vi "Teleop.vi"(10 "Match Info":T1={"Autonomous Elapsed Seconds"=0.0, "TeleOp Elapsed Seconds"=0.0, "Disabled Elapsed Seconds"=0.0, "Visited Autonomous"=FALSE, "Visited TeleOp"=FALSE, "Visited Disabled"=FALSE, "Autonomous Settings"={"Autonomous Style"=enum."Independent", "VI Refnum"=refnum}}, 11 "Call Context":T2) -> ()   [LabVIEW 2015]
doc: "This VI is called for each TeleOp packet received from the DS where the robot is not disabled. It is often used to read from the joysticks and update I/O or to update setpoints for timed control loops. It should complete and return within 20 milliseconds or it may miss DS packets."
uses:
  <vilib>/Rock Robotics/WPI/DriverStation/WPI_DriverStationDerivedRobotMode.ctl
  <vilib>/Rock Robotics/WPI/DriverStation/WPI_DriverStationMatch Info.ctl
  <vilib>/Rock Robotics/WPI/Solenoid/WPI_SolenoidValue.ctl
  <vilib>/Rock Robotics/WPI/Utilities/WPI_GetSetVariantRefNum.vi
  Robot Global Data.vi
  <vilib>/Rock Robotics/Network Tables/NT Write Boolean.vi
  <vilib>/Rock Robotics/Network Tables/NT Write Numeric Array.vi
  <vilib>/Rock Robotics/Network Tables/NT Read Boolean.vi
  <vilib>/Rock Robotics/Network Tables/NT Read Number.vi
  <vilib>/Rock Robotics/WPI/Solenoid/WPI_SolenoidSetEnum.vi
panel:
  out "Sample Slider 0":dbl(slide) scale=0.0..5.0
  out "Sample Boolean 1":bool
  out "Sample Boolean 0":bool
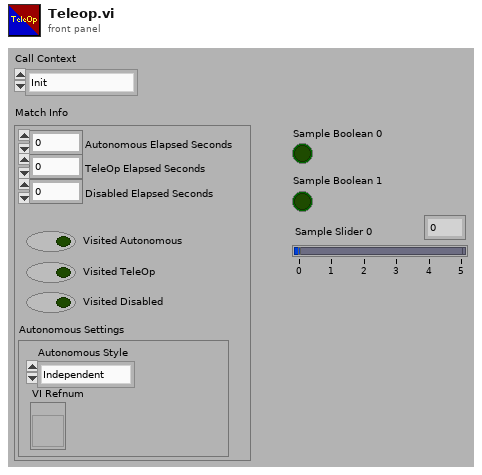
[diagram p1: front panel]
types:
  T1 = typedef "WPI_DriverStationMatch Info.ctl" = cluster{"Autonomous Elapsed Seconds":dbl, "TeleOp Elapsed Seconds":dbl, "Disabled Elapsed Seconds":dbl, "Visited Autonomous":bool, "Visited TeleOp":bool, "Visited Disabled":bool, "Autonomous Settings":cluster{"Autonomous Style":enum16{"Iterative", "Independent"}, "VI Refnum":refnum<vi>}}
  T2 = typedef "WPI_DriverStationDerivedRobotMode.ctl" = enum16{"Init", "Execute", "Stop"}
  T3 = typedef "WPI_SolenoidValue.ctl" = enum16{"Off", "On", "Forward", "Reverse"}
  T4 = typedef "WPI_JoystickDevRef.ctl" = cluster{"Device":T5}
  T5 = typedef "WPI_JoystickDeviceEnum.ctl" = enum16{"USB 0", "USB 1", "USB 2", "USB 3", "USB 4", "USB 5"}
  T6 = cluster{"Buttons[0]":bool, "Buttons[1]":bool, "Buttons[2]":bool, "Buttons[3]":bool, "Buttons[4]":bool, "Buttons[5]":bool, "Buttons[6]":bool, "Buttons[7]":bool, "Buttons[8]":bool}
  T7 = typedef "WPI_DigitalInputDevRef.ctl" = cluster{"DevStatus":errorcluster, "DIO Channel":T8}
  T8 = typedef "FPGA_DIOChannel.ctl" = enum8{"DIO 0", "DIO 1", "DIO 2", "DIO 3", "DIO 4", "DIO 5", "DIO 6", "DIO 7", "DIO 8", "DIO 9", "DIO MXP 0", "DIO MXP 1", "DIO MXP 2", "DIO MXP 3", "DIO MXP 4", "DIO MXP 5", "DIO MXP 6", "DIO MXP 7", "DIO MXP 8", "DIO MXP 9", "DIO MXP 10", "DIO MXP 11", "DIO MXP 12", "DIO MXP 13", "DIO MXP 14", "DIO MXP 15", "Invalid"}
  T9 = typedef "WPI_RobotDriveDevRef.ctl" = cluster{"DevStatus":errorcluster, "Motors[]":T10[], "Square Inputs":bool, "Max Output":dbl}
  T10 = typedef "WPI_MotorControlDeviceRef.ctl" = cluster{"DeviceStatus":errorcluster, "Type":T11, "PWM":cluster{"PWM Channel":T12, "DeadBand":T13}, "CAN":cluster{"Device Number":u8, "Control Mode":T14, "Semaphore":T15, "Max Vout":dbl, "TalonSRX Control Mode":T16}, "Invert":bool}
  T11 = typedef "WPI_MotorControlType.ctl" = enum16{"PWM", "CAN", "CANTalonSRX"}
  T12 = typedef "FPGA_DIOPWMChannel.ctl" = enum8{"PWM 0", "PWM 1", "PWM 2", "PWM 3", "PWM 4", "PWM 5", "PWM 6", "PWM 7", "PWM 8", "PWM 9", "PWM MXP 0", "PWM MXP 1", "PWM MXP 2", "PWM MXP 3", "PWM MXP 4", "PWM MXP 5", "PWM MXP 6", "PWM MXP 7", "PWM MXP 8", "PWM MXP 9", "Invalid"}
  T13 = typedef "WPI_PWMDeadband.ctl" = cluster{"Name":string, "maxPositivePwm":i32, "minPositivePwm":i32, "centerPwm":i32, "maxNegativePwm":i32, "minNegativePwm":i32, "angularRange":u16}
  T14 = typedef "WPI_CANJaguar_ControlMode.ctl" = enum8{"Percent VBus", "Current", "Speed", "Position", "Voltage"}
  T15 = typedef "Semaphore RefNum" = refnum<k1>
  T16 = typedef "WPI_CANTalonSRX_APIControlMode.ctl" = enum8{"Percent VBus", "Speed", "Position", "Slave", "Unchanged / Invalid", "Voltage Compensation", "Current", "Motion Profile"}
  T17 = typedef "WPI_SolenoidDevRef.ctl" = cluster{"DevStatus":errorcluster, "Pneumatics Control Module":u8, "Forward Solenoid Channel":T18, "Reverse Solenoid Channel":T18}
  T18 = typedef "WPI_SolenoidChannel.ctl" = enum8{"Solenoid 0", "Solenoid 1", "Solenoid 2", "Solenoid 3", "Solenoid 4", "Solenoid 5", "Solenoid 6", "Solenoid 7", "Invalid"}
  T19 = typedef "WPI_ServoDeviceRef.ctl" = cluster{"DeviceStatus":errorcluster, "PWM Channel":T12, "DeadBand":T13}
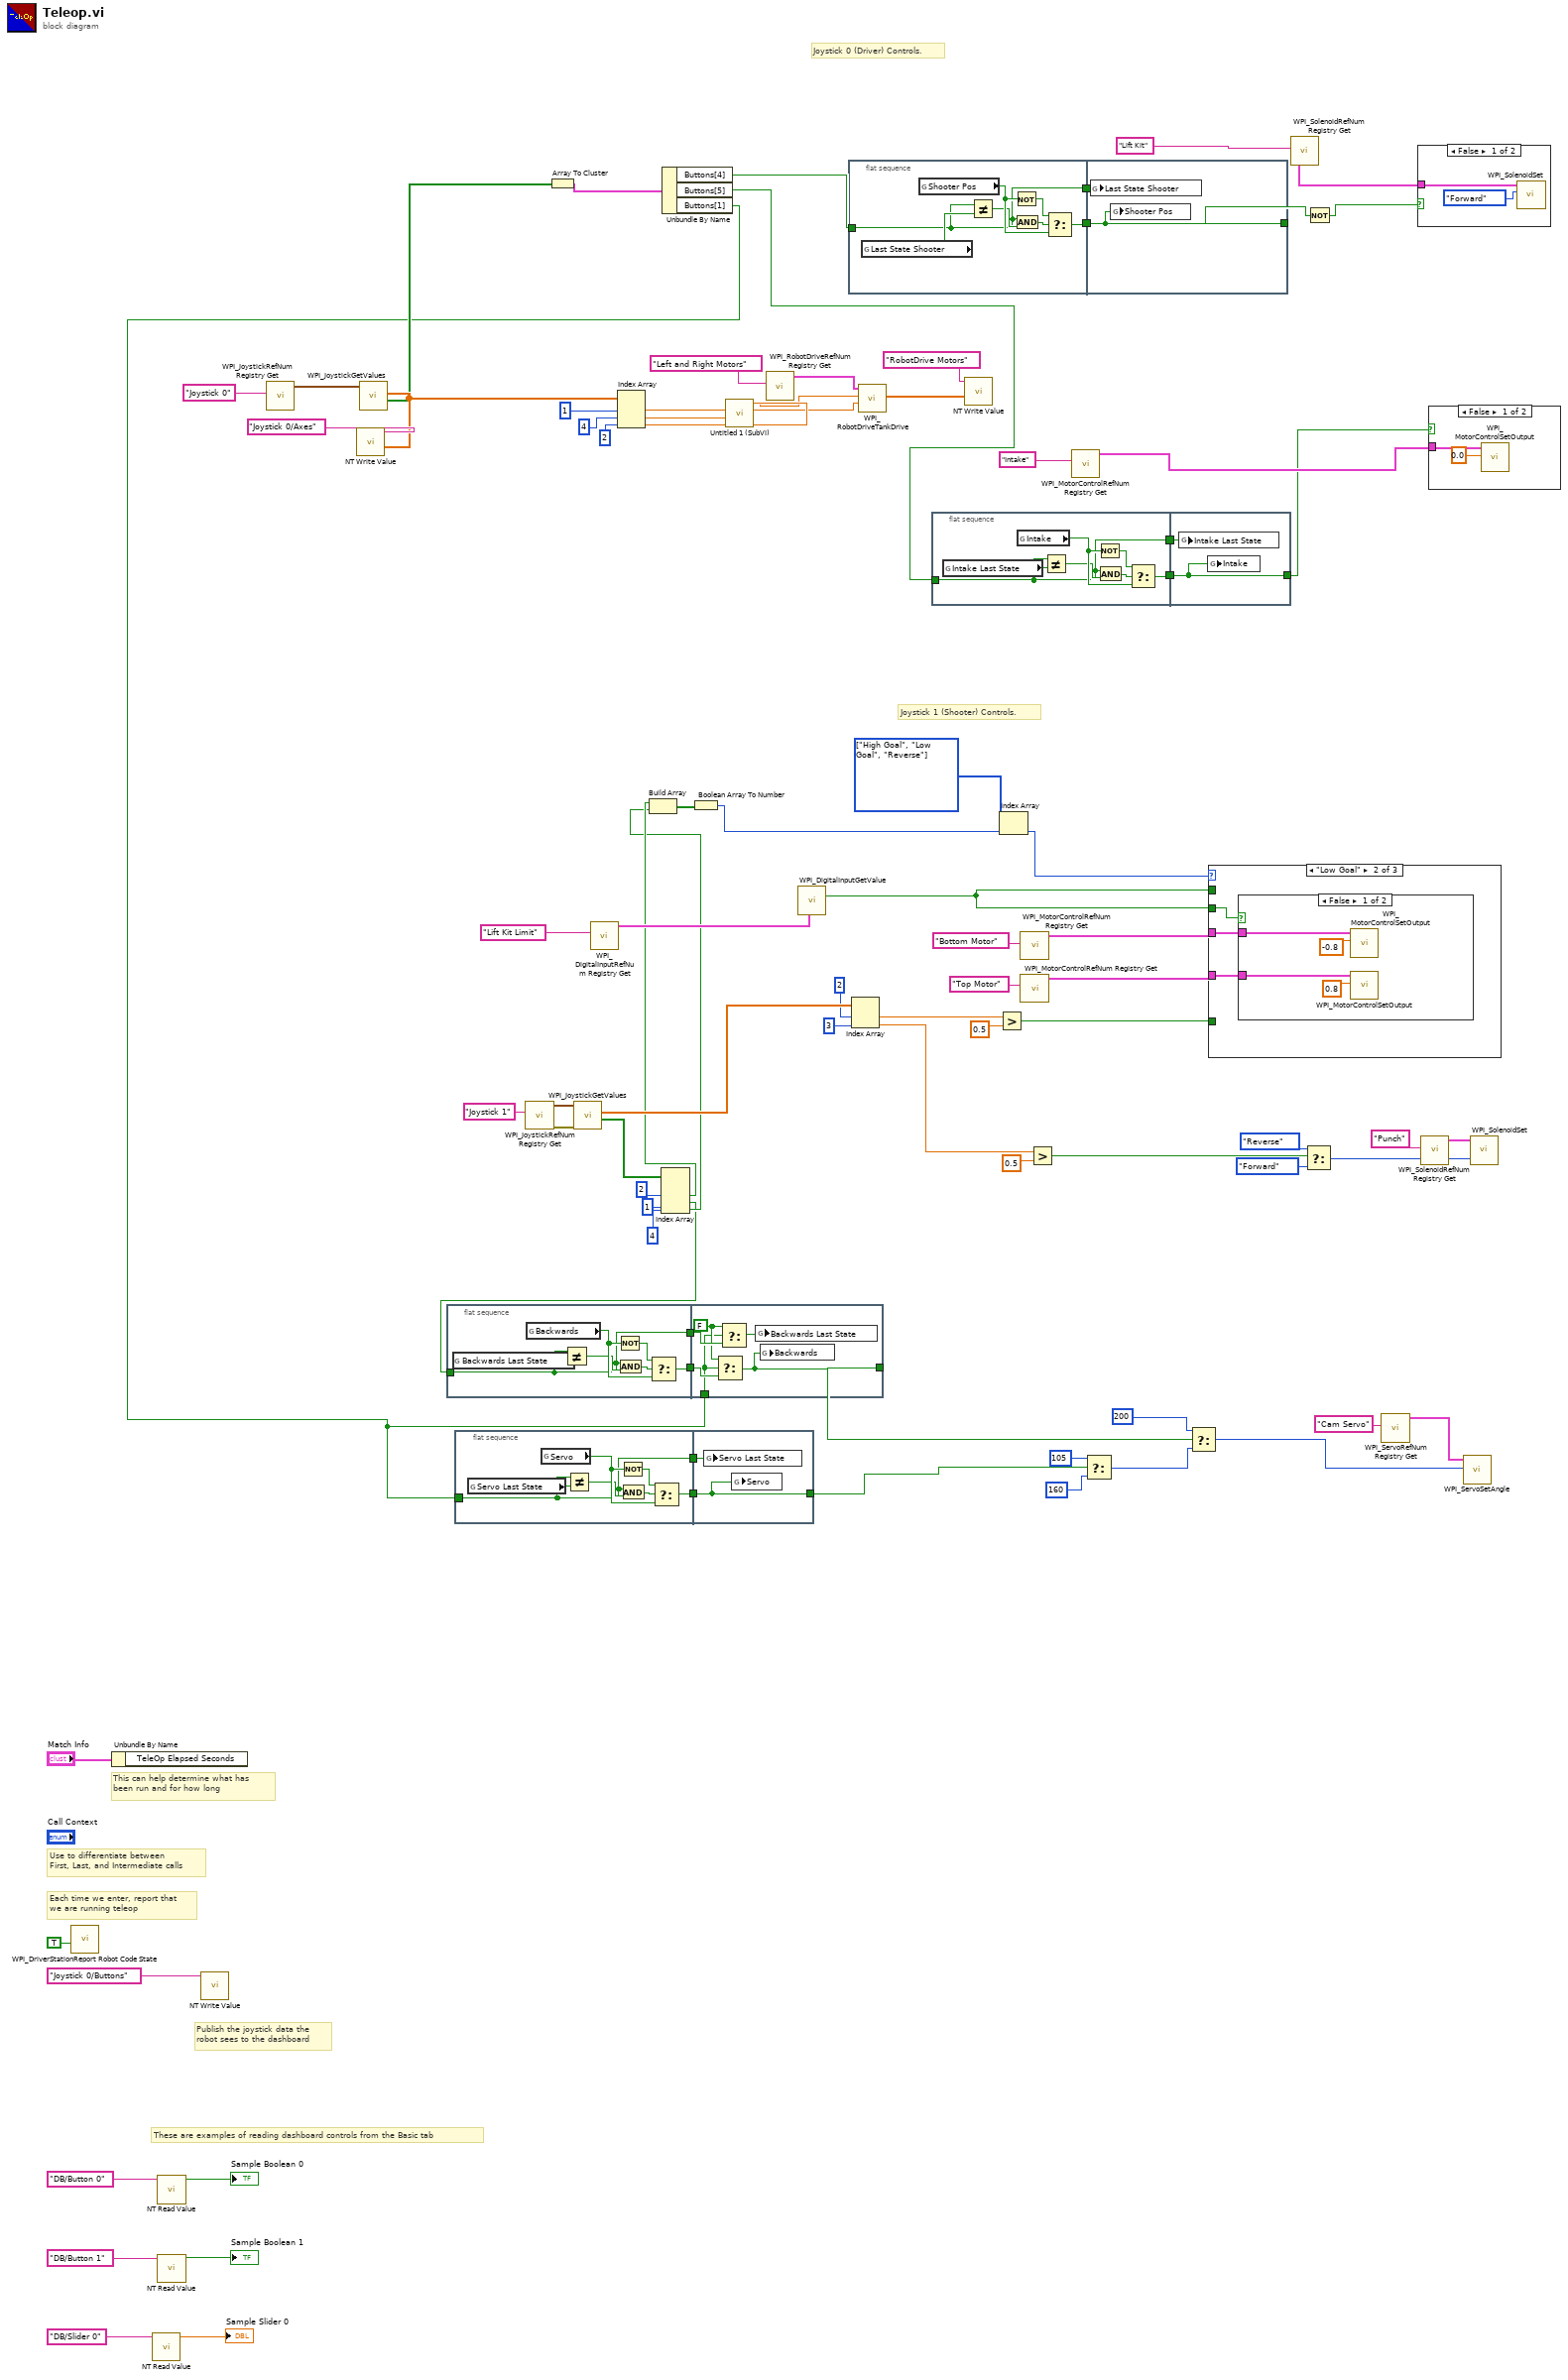
[diagram p0: block diagram]
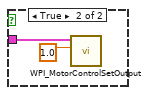
[diagram p2: hidden frame]
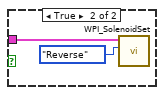
[diagram p3: hidden frame]
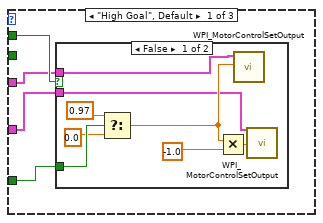
[diagram p4: hidden frame]
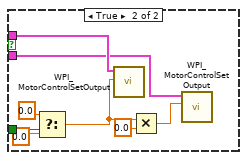
[diagram p5: hidden frame]
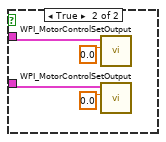
[diagram p6: hidden frame]
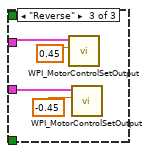
[diagram p7: hidden frame]
diagram:
  w29 = enum16{"High Goal", "Low Goal", "Reverse", ""}[] [enum."High Goal", enum."Low Goal", enum."Reverse"] items=["High Goal", "Low Goal", "Reverse", ""] ("array")
  # "Joystick 1 (Shooter) Controls."
  # "Joystick 0 (Driver) Controls."
  # "These are examples of reading dashboard controls from the Basic tab"
  # "Publish the joystick data the\nrobot sees to the dashboard"
  # "Each time we enter, report that\nwe are running teleop"
  # "Use to differentiate between\nFirst, Last, and Intermediate calls"
  # "This can help determine what has\nbeen run and for how long"
  n1 = call <vilib>:"WPI_DriverStationReport Robot Code State.vi"("TeleOp"=TRUE ("Autonomous")) -> ()  [unwired: 10 in, 1 out]
  n2 = Unbundle By Name("Match Info") -> ()  [unwired: 1 out]
  n3 = call-poly <vilib>:"NT Read Value.vi"("Name"="DB/Slider 0" ("refnum name")) -> ("Numeric"=→"Sample Slider 0":dbl)  [unwired: 9 in, 1 out]
  n4 = call-poly <vilib>:"NT Read Value.vi"("Name"="DB/Button 0" ("refnum name")) -> ("Boolean"=→"Sample Boolean 0":bool)  [unwired: 9 in, 1 out]
  n5 = call-poly <vilib>:"NT Read Value.vi"("Name"="DB/Button 1" ("refnum name")) -> ("Boolean"=→"Sample Boolean 1":bool)  [unwired: 9 in, 1 out]
  n6 = call-poly <vilib>:"NT Write Value.vi"("Name"="Joystick 0/Buttons") -> ()  [unwired: 10 in, 1 out]
  n7 = call <vilib>:"WPI_JoystickRefNum Registry Get.vi"("refnum name"="Joystick 0") -> ("JoystickDevRef"=w87:T4)  [unwired: 1 in, 9 out]
  n8 = call <vilib>:"WPI_JoystickGetValues.vi"("JoystickDevRef"=w87) -> ("Buttons"=w74:bool[], "Axes"=w83:dbl[])  [unwired: 6 in, 3 out]
  n9 = call-poly <vilib>:"NT Write Value.vi"("Numeric Array"=w83, "Name"="Joystick 0/Axes") -> ()  [unwired: 9 in, 1 out]
  n10 = flat-sequence {
    tunnel: w9 -> [w90]
    tunnel: [w94] -> w11
    tunnel: [w90] -> w10
    tunnel: w11 -> [w99]
    tunnel: [w100] -> w8
    tunnel: w10 -> [w101]
    tunnel: w1 -> [w97]
    frame #0 {
      n11 = global read "Robot Global Data.vi" "Backwards Last State"() -> (w93:bool)
      n12 = global read "Robot Global Data.vi" "Backwards"() -> (w95:bool)
      n13 = Not Equal?(x=w90, y=w93) -> (x != y?=w91:bool)
      n14 = Not(x=w95) -> (.not. x?=w96:bool)
      n15 = And(x=w90, y=w91) -> (x .and. y?=w92:bool)
      n16 = Select(t=w96, s=w92, f=w95) -> (s? t:f=w94:bool)
    }
    frame #1 {
      w98 = FALSE ("t")
      n17 = Select(t=w98, s=w97, f=w99) -> (s? t:f=w100:bool)
      n18 = Select(t=w98, s=w97, f=w101) -> (s? t:f=w102:bool)
      n19 = global write "Robot Global Data.vi" "Backwards Last State"(w102) -> ()
      n20 = global write "Robot Global Data.vi" "Backwards"(w100) -> ()
    }
  }
  n21 = flat-sequence {
    tunnel: w1 -> [w103]
    tunnel: [w107] -> w18
    tunnel: [w103] -> w17
    tunnel: w18 -> [w111]
    tunnel: [w111] -> w7
    tunnel: w17 -> [w110]
    frame #0 {
      n22 = global read "Robot Global Data.vi" "Servo Last State"() -> (w106:bool)
      n23 = global read "Robot Global Data.vi" "Servo"() -> (w108:bool)
      n24 = Not Equal?(x=w103, y=w106) -> (x != y?=w104:bool)
      n25 = Not(x=w108) -> (.not. x?=w109:bool)
      n26 = And(x=w103, y=w104) -> (x .and. y?=w105:bool)
      n27 = Select(t=w109, s=w105, f=w108) -> (s? t:f=w107:bool)
    }
    frame #1 {
      n28 = global write "Robot Global Data.vi" "Servo Last State"(w110) -> ()
      n29 = global write "Robot Global Data.vi" "Servo"(w111) -> ()
    }
  }
  n30 = call <vilib>:"WPI_JoystickRefNum Registry Get.vi"("refnum name"="Joystick 1") -> ("error out"=w69:errorcluster, "JoystickDevRef"=w68:T4)  [unwired: 1 in, 8 out]
  n31 = Array To Cluster(array=w74) -> (cluster=w76:T6)
  n32 = call <vilib>:"WPI_JoystickGetValues.vi"("error in (no error)"=w69, "JoystickDevRef"=w68) -> ("Buttons"=w54:bool[], "Axes"=w67:dbl[])  [unwired: 5 in, 3 out]
  n33 = call <vilib>:"WPI_DigitalInputRefNum Registry Get.vi"("refnum name"="Lift Kit Limit") -> ("DigitalInputDevRef"=w57:T7)  [unwired: 9 in, 1 out]
  n34 = Index Array(array=w83, index #1=1 ("index"), index #2=4 ("index"), index #3=2 ("index")) -> (element #1=w61:dbl, element #2=w62:dbl, element #3=w60:dbl)
  n35 = Index Array(array=w54, index #2=2 ("index"), index #3=1 ("index"), index #4=4 ("index")) -> (element #2=w36:bool, element #3=w9:bool, element #4=w35:bool)  [unwired: 1 in, 1 out]
  n36 = Build Array(w36, w35) -> (w27:bool[])
  n37 = Unbundle By Name(w76) -> ("Buttons[4]"=w25:bool, "Buttons[5]"=w19:bool, "Buttons[1]"=w1:bool)
  n38 = Boolean Array To Number(Boolean array=w27) -> (number=w26:u32)
  n39 = call "Untitled 1 (SubVI).vi"("upper limit 2"=w62, "upper limit"=w61, "Throttle"=w60) -> ("Numeric 2"=w47:dbl, "Numeric"=w48:dbl)  [unwired: 7 in]
  n40 = call <vilib>:"WPI_RobotDriveRefNum Registry Get.vi"("refnum name"="Left and Right Motors") -> ("RobotDriveDevRef"=w46:T9)  [unwired: 1 in, 9 out]
  n41 = call <vilib>:"WPI_DigitalInputGetValue.vi"("DigitalInputDevRef"=w57) -> ("Value"=w55:bool)  [unwired: 8 in, 2 out]
  n42 = flat-sequence {
    tunnel: w25 -> [w112]
    tunnel: [w116] -> w24
    tunnel: [w112] -> w23
    tunnel: w24 -> [w120]
    tunnel: [w120] -> w16
    tunnel: w23 -> [w119]
    frame #0 {
      n43 = global read "Robot Global Data.vi" "Last State Shooter"() -> (w115:bool)
      n44 = global read "Robot Global Data.vi" "Shooter Pos"() -> (w117:bool)
      n45 = Not Equal?(x=w112, y=w115) -> (x != y?=w113:bool)
      n46 = Not(x=w117) -> (.not. x?=w118:bool)
      n47 = And(x=w112, y=w113) -> (x .and. y?=w114:bool)
      n48 = Select(t=w118, s=w114, f=w117) -> (s? t:f=w116:bool)
    }
    frame #1 {
      n49 = global write "Robot Global Data.vi" "Last State Shooter"(w119) -> ()
      n50 = global write "Robot Global Data.vi" "Shooter Pos"(w120) -> ()
    }
  }
  n51 = Index Array(array=w67, index #1=2 ("index"), index #2=3 ("index")) -> (element #1=w66:dbl, element #2=w32:dbl)
  n52 = call <vilib>:"WPI_RobotDriveTankDrive.vi"("Right axis value"=w47, "Left axis value"=w48, "RobotDriveDevRef"=w46) -> ("Motor Values"=w71:dbl[])  [unwired: 6 in, 2 out]
  n53 = flat-sequence {
    tunnel: w19 -> [w121]
    tunnel: [w125] -> w22
    tunnel: [w121] -> w21
    tunnel: w22 -> [w129]
    tunnel: [w129] -> w20
    tunnel: w21 -> [w128]
    frame #0 {
      n54 = global read "Robot Global Data.vi" "Intake Last State"() -> (w124:bool)
      n55 = global read "Robot Global Data.vi" "Intake"() -> (w126:bool)
      n56 = Not Equal?(x=w121, y=w124) -> (x != y?=w122:bool)
      n57 = Not(x=w126) -> (.not. x?=w127:bool)
      n58 = And(x=w121, y=w122) -> (x .and. y?=w123:bool)
      n59 = Select(t=w127, s=w123, f=w126) -> (s? t:f=w125:bool)
    }
    frame #1 {
      n60 = global write "Robot Global Data.vi" "Intake Last State"(w128) -> ()
      n61 = global write "Robot Global Data.vi" "Intake"(w129) -> ()
    }
  }
  n62 = call-poly <vilib>:"NT Write Value.vi"("Numeric Array"=w71, "Name"="RobotDrive Motors") -> ()  [unwired: 9 in, 1 out]
  n63 = Greater?(x=w66, y=0.5) -> (0:w65:bool)
  n64 = Index Array(array=w29, index=w26) -> (element=w28:enum16{"High Goal", "Low Goal", "Reverse", ""})
  n65 = call <vilib>:"WPI_MotorControlRefNum Registry Get.vi"("refnum name"="Bottom Motor") -> ("MotorControlDevRef"=w39:T10)  [unwired: 9 in, 1 out]
  n66 = call <vilib>:"WPI_MotorControlRefNum Registry Get.vi"("refnum name"="Top Motor") -> ("MotorControlDevRef"=w38:T10)  [unwired: 9 in, 1 out]
  n67 = Greater?(x=w32, y=0.5) -> (0:w30:bool)
  n68 = call <vilib>:"WPI_MotorControlRefNum Registry Get.vi"("refnum name"="Intake") -> ("MotorControlDevRef"=w50:T10)  [unwired: 9 in, 1 out]
  n69 = Select(t=105, s=w7, f=160 ("Angle")) -> (s? t:f=w3:i32)
  n70 = Select(t=200 ("Angle"), s=w8, f=w3) -> (s? t:f=w2:i32)
  n71 = case shown="\"Low Goal\"" w28 {
    tunnel: w65 -> [w133 _ _]
    tunnel: w55 -> [_ w152 _]
    tunnel: w55 -> [w132 _ _]
    tunnel: w39 -> [w131 w151 w162]
    tunnel: w38 -> [w130 w150 w161]
    frame "High Goal", Default {
      n72 = case shown="False" w132 {
        tunnel: w133 -> [w140 w149]
        tunnel: w131 -> [w134 w143]
        tunnel: w130 -> [w135 w142]
        frame False {
          n73 = Select(t=0.97, s=w140, f=0.0) -> (s? t:f=w139:dbl)
          n74 = Multiply(x=w139, y=-1.0) -> (x*y=w141:dbl)
          n75 = call <vilib>:"WPI_MotorControlSetOutput.vi"("Output"=w139, "MotorControlDevRef"=w134) -> ()  [unwired: 7 in, 3 out]
          n76 = call <vilib>:"WPI_MotorControlSetOutput.vi"("Output"=w141, "MotorControlDevRef"=w135) -> ()  [unwired: 7 in, 3 out]
        }
        frame True {
          n77 = Select(t=0.0, s=w149, f=0.0) -> (s? t:f=w148:dbl)
          n78 = call <vilib>:"WPI_MotorControlSetOutput.vi"("Output"=w148, "MotorControlDevRef"=w143) -> ()  [unwired: 7 in, 3 out]
          n79 = Multiply(x=w148, y=0.0) -> (x*y=w146:dbl)
          n80 = call <vilib>:"WPI_MotorControlSetOutput.vi"("Output"=w146, "MotorControlDevRef"=w142) -> ()  [unwired: 7 in, 3 out]
        }
      }
    }
    frame "Low Goal" {
      n81 = case shown="False" w152 {
        tunnel: w151 -> [w154 w157]
        tunnel: w150 -> [w153 w158]
        frame False {
          n82 = call <vilib>:"WPI_MotorControlSetOutput.vi"("Output"=-0.8, "MotorControlDevRef"=w154) -> ()  [unwired: 7 in, 3 out]
          n83 = call <vilib>:"WPI_MotorControlSetOutput.vi"("Output"=0.8, "MotorControlDevRef"=w153) -> ()  [unwired: 7 in, 3 out]
        }
        frame True {
          n84 = call <vilib>:"WPI_MotorControlSetOutput.vi"("Output"=0.0, "MotorControlDevRef"=w157) -> ()  [unwired: 7 in, 3 out]
          n85 = call <vilib>:"WPI_MotorControlSetOutput.vi"("Output"=0.0, "MotorControlDevRef"=w158) -> ()  [unwired: 7 in, 3 out]
        }
      }
    }
    frame "Reverse" {
      n86 = call <vilib>:"WPI_MotorControlSetOutput.vi"("Output"=0.45, "MotorControlDevRef"=w162) -> ()  [unwired: 7 in, 3 out]
      n87 = call <vilib>:"WPI_MotorControlSetOutput.vi"("Output"=-0.45, "MotorControlDevRef"=w161) -> ()  [unwired: 7 in, 3 out]
    }
  }
  n88 = call <vilib>:"WPI_SolenoidRefNum Registry Get.vi"("refnum name"="Lift Kit") -> ("SolenoidDevRef"=w72:T17)  [unwired: 9 in, 1 out]
  n89 = Select(t=WPI_SolenoidValue."Reverse" ("Value"), s=w30, f=WPI_SolenoidValue."Forward" ("Value")) -> (s? t:f=w52:T3)
  n90 = Not(x=w16) -> (.not. x?=w15:bool)
  n91 = call <vilib>:"WPI_ServoRefNum Registry Get.vi"("refnum name"="Cam Servo") -> ("ServoDeviceRef"=w12:T19)  [unwired: 9 in, 1 out]
  n92 = case shown="False" w15 {
    tunnel: w72 -> [w166 w168]
    frame False {
      n93 = call-poly <vilib>:"WPI_SolenoidSet.vi"("Value"=WPI_SolenoidValue."Forward", "SolenoidDevRef"=w166) -> ()  [unwired: 8 in, 2 out]
    }
    frame True {
      n94 = call-poly <vilib>:"WPI_SolenoidSet.vi"("Value"=WPI_SolenoidValue."Reverse", "SolenoidDevRef"=w168) -> ()  [unwired: 8 in, 2 out]
    }
  }
  n95 = call <vilib>:"WPI_SolenoidRefNum Registry Get.vi"("refnum name"="Punch") -> ("SolenoidDevRef"=w53:T17)  [unwired: 9 in, 1 out]
  n96 = case shown="False" w20 {
    tunnel: w50 -> [w170 w172]
    frame False {
      n97 = call <vilib>:"WPI_MotorControlSetOutput.vi"("Output"=0.0, "MotorControlDevRef"=w170) -> ()  [unwired: 7 in, 3 out]
    }
    frame True {
      n98 = call <vilib>:"WPI_MotorControlSetOutput.vi"("Output"=1.0, "MotorControlDevRef"=w172) -> ()  [unwired: 7 in, 3 out]
    }
  }
  n99 = call <vilib>:"WPI_ServoSetAngle.vi"("Angle"=w2, "ServoDeviceRef"=w12) -> ()  [unwired: 8 in, 2 out]
  n100 = call-poly <vilib>:"WPI_SolenoidSet.vi"("Value"=w52, "SolenoidDevRef"=w53) -> ()  [unwired: 8 in, 2 out]
